vi "Create.vi"(8 "error in (no error)":errorcluster, 10 "I2C #":T1=-1) -> (0 "error out":errorcluster, 3 "I2C out":refnum<class "I2C.lvclass">)   [LabVIEW 2024, in "CTI.lvlib" / "I2C.lvclass"]
uses:
  I2C.lvclass
  I2C Number.ctl
  I2C.lvclass/I2C.ctl
  CTI.lvlib
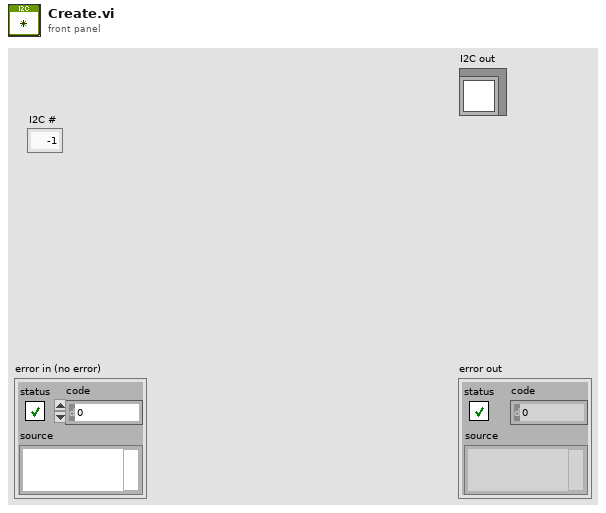
[diagram p1: front panel]
types:
  T1 = typedef "CTI.lvlib/I2C Number.ctl" = i8
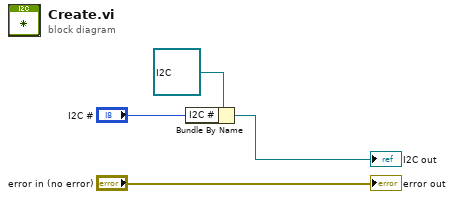
[diagram p0: block diagram]
diagram:
  n1 = Bundle By Name(cluster=refnum<class "I2C.lvclass"> refnum ("I2C in"), "I2C #"="I2C #") -> (→"I2C out":refnum<class "I2C.lvclass">)
  "error out" <- "error in (no error)"
